vi "getAttributeTreeUnitTooltip_action.vi"(0 "HGF_IMAQDevice":refnum<class "HGF_IMAQDevice.lvclass">, 1 "Tree Control In":refnum<vi>, 2 "Force update?":bool, 3 "Tab Control Ref In":T1, 5 "error in (no error)":errorcluster) -> (14 "dup HGF_IMAQDevice":refnum<class "HGF_IMAQDevice.lvclass">, 15 "Tree Control Out":refnum<vi>, 16 "Units":string, 17 "Tooltip":string, 19 "error out":errorcluster)   [LabVIEW 2014, in "HGF_IMAQ.lvlib" / "HGF_IMAQDevice.lvclass"]
doc: "This is the override VI to read cameras attribute unit and tooltip."
uses:
  HGF_IMAQDevice.lvclass
  HGF_Auxiliary/HGF_Auxiliary.lvlib
  HGF_Auxiliary/Severity.ctl
  HGF_Auxiliary/ErrorCode.ctl
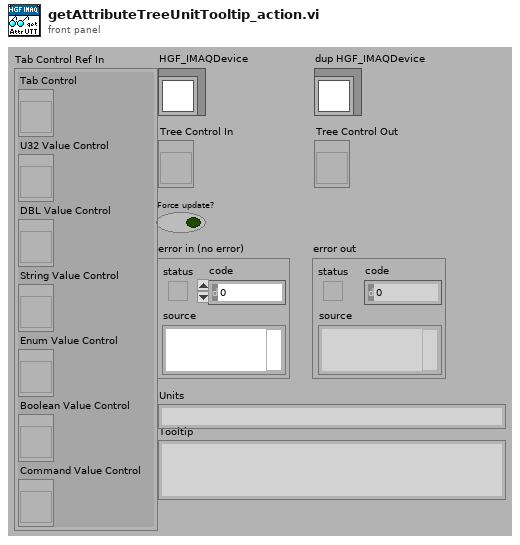
[diagram p1: front panel]
types:
  T1 = cluster{"Tab Control":refnum<vi>, "U32 Value Control":refnum<vi>, "DBL Value Control":refnum<vi>, "String Value Control":refnum<vi>, "Enum Value Control":refnum<vi>, "Boolean Value Control":refnum<vi>, "Command Value Control":refnum<vi>}
  T2 = typedef "HGF_Auxiliary.lvlib/ErrorCode.ctl" = enum32{"No error", "Function not supported.", "This VI is for friends only.", "Reference object aready exisits.", "Parameter out of range.", "Not a rendezvous.", "Invalid notifier reference.", "Invalid queue reference.", "Self-Test not supported.", "Reset not supported.", "IDN query not supported.", "Error query not supported.", "Incorrect addressee.", "Object already exists.", "No class name specified", "Driver not supported", "Attribute is not writable"}
  T3 = typedef "HGF_Auxiliary.lvlib/Severity.ctl" = enum16{"Info", "Warning", "Fault", "Error", "Fatal"}
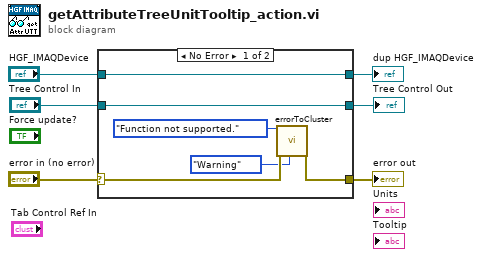
[diagram p0: block diagram]
diagram:
  n1 = case shown="No Error" "error in (no error)" {
    selector: "error in (no error)" -> [w12 w13]
    tunnel: [w11 w13] -> w5
    tunnel: [w8 w14] -> w3
    tunnel: "HGF_IMAQDevice" -> [w8 w14]
    tunnel: "Tree Control In" -> [w7 _]
    tunnel: [w7 _] -> w1
    frame No Error {
      n2 = call "errorToCluster.vi"("error code"=ErrorCode."Function not supported.", "error in (no error)"=w12, "severity (Error)"=Severity."Warning") -> ("error out"=w11:errorcluster)  [unwired: 16 in]
    }
    frame Error {
    }
  }
  "error out" <- w5
  "dup HGF_IMAQDevice" <- w3
  "Tree Control Out" <- w1
